vi "DAQ_Controls_Integration.vi"() -> ()   [LabVIEW 2017]
uses:
  <vilib>/MakerHub/LINX/Public/Peripherals/Digital/Digital Write N Chans.vi
  <vilib>/MakerHub/LINX/Private/Local IO/LinxDigitalWrite.vi
  <vilib>/MakerHub/LINX/Public/Utilities/Check Channel.vi
  <vilib>/MakerHub/LINX/Public/Utilities/Open Serial.vi
  <vilib>/MakerHub/LINX/Private/Utilties/Generate Error.vi
  <vilib>/Waveform/WDTOps.llb/WDT Append Waveforms DBL.vi
  <vilib>/MakerHub/LINX/LMH-LINX.lvlib
panel:
  in  "Stop Button":bool
  in  "MANUAL CONTROLS":bool[](array[boolean])
  out "Loop Rate (Hz)":u32
  in  "CHANNELS":u8[](array[numeric])
  in  "Serial Port":refnum<visa-resource-name>
  in  "stop":bool
  out "Waveform Chart":waveform(dbl)(graph)
  in  "Recording Data":bool
  out "Waveform Chart 2":waveform(dbl)(graph)
  out "Numeric":dbl
  out "Numeric 2":dbl
  out "Difference between signals 1 & 2":dbl
  out "Waveform Chart 3":waveform(dbl)(graph)
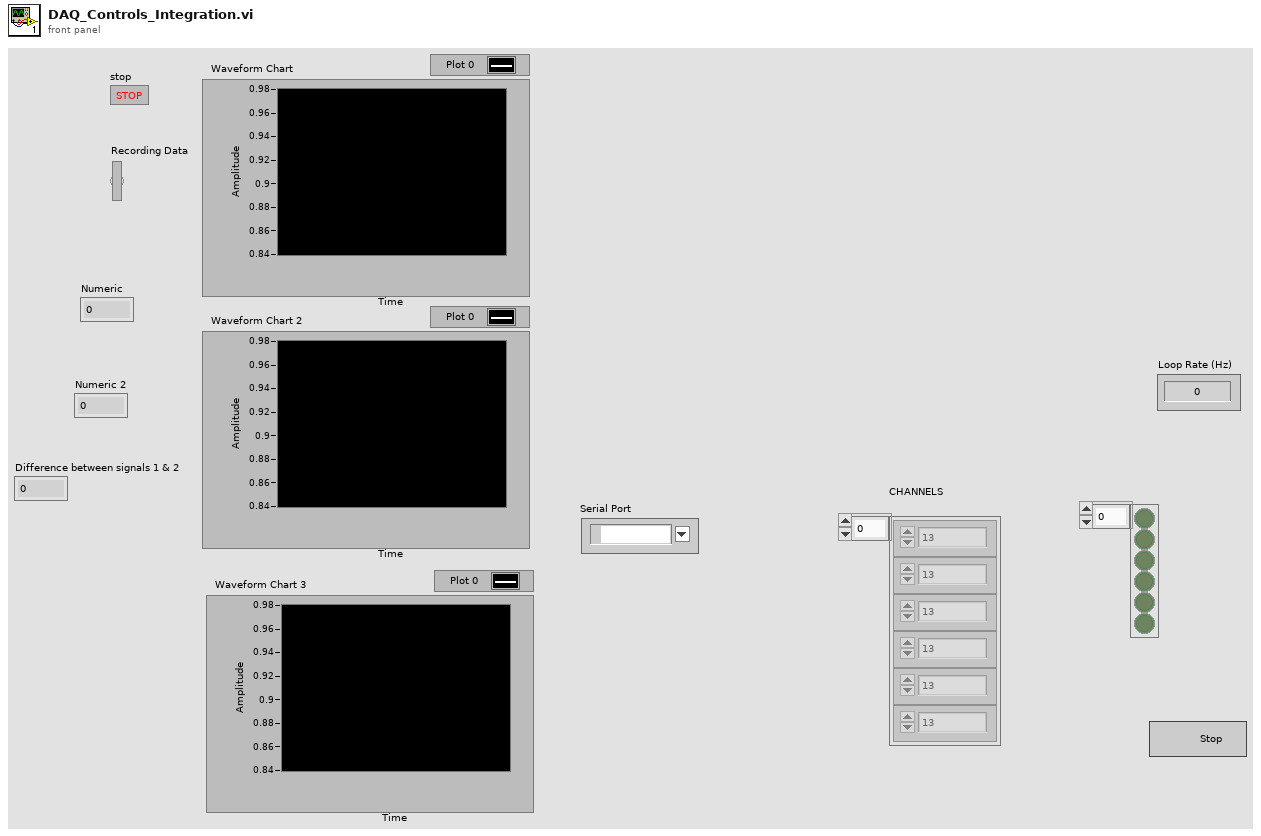
[diagram p1: front panel]
types:
  T1 = typedef "LMH-LINX.lvlib/LINX Ref.ctl" = cluster{"IO":T2, "Interface":T3, "LINX Device Config":T4}
  T2 = typedef "LMH-LINX.lvlib/Platform.ctl" = enum16{"Remote", "Local"}
  T3 = typedef "LMH-LINX.lvlib/Interface.ctl" = enum16{"Serial", "TCP"}
  T4 = typedef "LMH-LINX.lvlib/Device.lvlib/LINX Device Config.ctl" = cluster{"Interface":T3, "COM Port":refnum<visa-resource-name>, "TCP Configuration":T5, "Device Family":u8, "Device ID":u8, "Device Name":string, "TCP Ref":refnum<k5>, "Channels":T6}
  T5 = typedef "LMH-LINX.lvlib/Device.lvlib/TCP Config.ctl" = cluster{"IP Address":string, "Port":u16}
  T6 = typedef "LMH-LINX.lvlib/Channels.ctl" = cluster{"DI":u8[], "DO":u8[], "AI":u8[], "AO":u8[], "PWM":u8[], "QE":u8[], "UART":u8[], "I2C 2":u8[], "SPI":u8[], "CAN":u8[], "Servo":u8[], "AI Ref (V)":dbl, "AI Resolution (Bits)":u8, "AO Ref (V)":dbl, "AO Resolution (Bits)":u8}
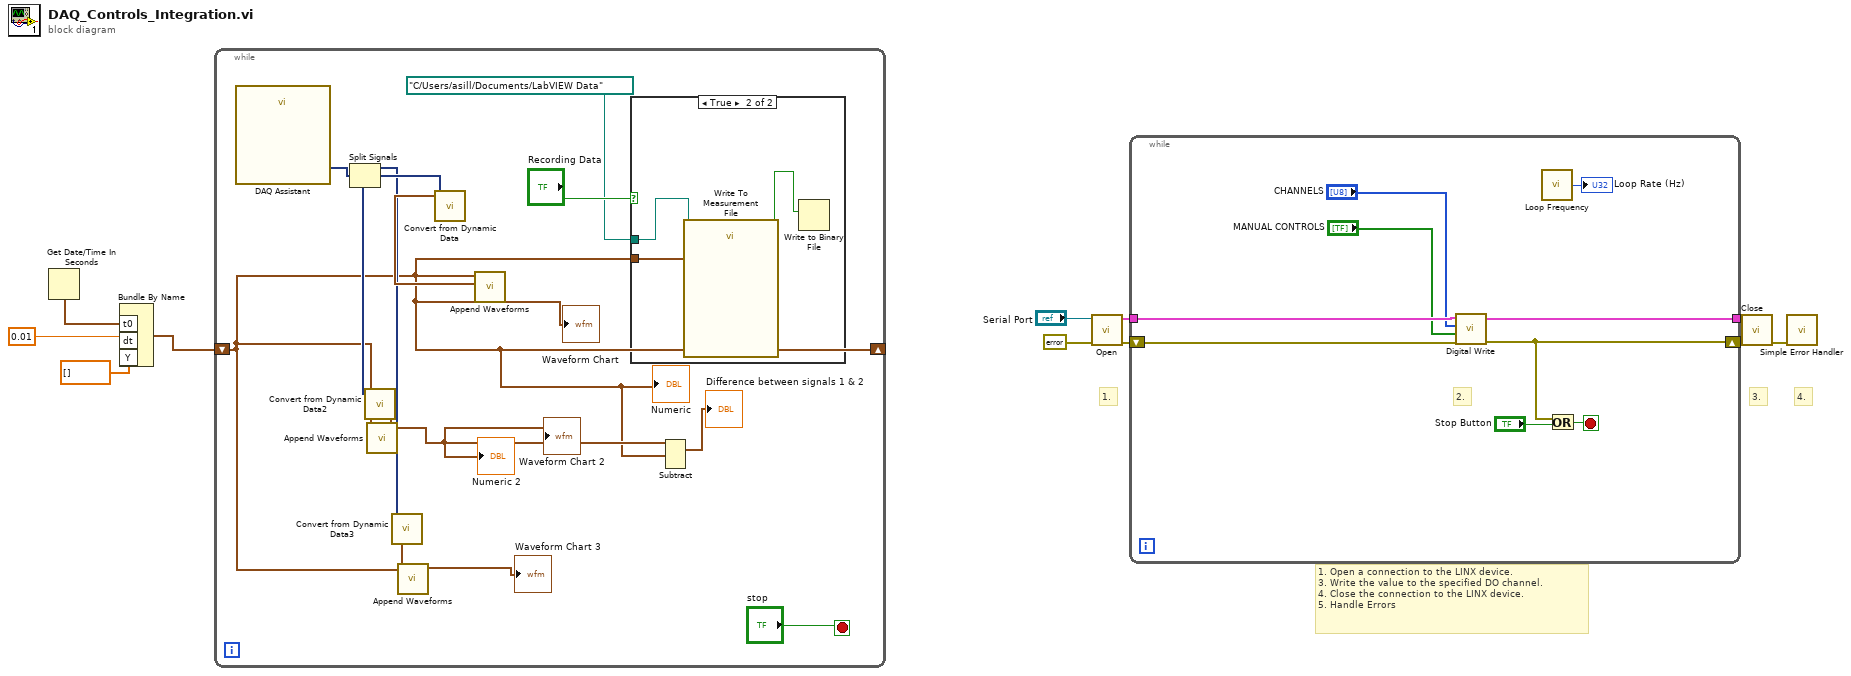
[diagram p0: block diagram]
diagram:
  # "1. Open a connection to the LINX device.\n3. Write the value to the specified DO channel.\n4. Close the connection to the LINX device.\n5. Handle Errors"
  # "4."
  # "3."
  # "1."
  n1 = Get Date/Time In Seconds() -> (seconds since 1Jan1904=w9:timestamp)
  n2 = Bundle By Name("t0"=w9, "dt"=0.01, "Y"=dbl[] []) -> (w10:waveform(dbl))  [unwired: 1 in]
  n3 = while {
    shift-right: [w17] -> _
    shift-left: w10 -> [w13]
    stop <- "stop" stop-if-true
    n4 = call "DAQ Assistant"() -> ("data"=w21:dynamicdata)  [unwired: 16 in, 3 out]
    n5 = Split Signals(w21) -> (w15:dynamicdata, w20:dynamicdata, w19:dynamicdata)  [unwired: 3 in]
    n6 = call "Convert from Dynamic Data2"("Dynamic Data Type"=w19) -> ("Waveform"=w22:waveform(dbl))  [unwired: 3 in]
    n7 = call-poly <vilib>:"Append Waveforms.vi"("waveform B"=w22, "waveform A"=w13) -> ("waveform out"=w18:waveform(dbl))  [unwired: 8 in, 1 out]
    "Waveform Chart 2" <- w18
    "Numeric 2" <- w18
    n8 = call "Convert from Dynamic Data3"("Dynamic Data Type"=w15) -> ("Waveform"=w14:waveform(dbl))  [unwired: 3 in]
    n9 = call-poly <vilib>:"Append Waveforms.vi"("waveform B"=w14, "waveform A"=w13) -> ("waveform out"=→"Waveform Chart 3":waveform(dbl))  [unwired: 8 in, 1 out]
    n10 = call "Convert from Dynamic Data"("Dynamic Data Type"=w20) -> ("Waveform"=w25:waveform(dbl))  [unwired: 3 in]
    n11 = call-poly <vilib>:"Append Waveforms.vi"("waveform B"=w25, "waveform A"=w13) -> ("waveform out"=w17:waveform(dbl))  [unwired: 8 in, 1 out]
    "Waveform Chart" <- w17
    "Numeric" <- w17
    n12 = case shown="True" "Recording Data" {
      tunnel: path "C:/Users/asill/Documents/LabVIEW Data" -> [_ w28]
      tunnel: w17 -> [_ w27]
      frame False {
      }
      frame True {
        n13 = call "Write To Measurement File"("Signals"=w27, "Filename"=w28) -> ("Saving Data"=w29:bool)  [unwired: 15 in, 2 out]
        n14 = Write to Binary File(data=w29) -> ()  [unwired: 5 in, 3 out]
      }
    }
    n15 = Subtract(1:w17, 2:w18) -> (0:→"Difference between signals 1 & 2":waveform(dbl))  [unwired: 1 in, 1 out]
  }
  n16 = call-poly <vilib>:"Open.vi"("Error In"=errorcluster {"status"=FALSE, "code"=0, "source"=""}, "Serial Port"="Serial Port") -> ("Error Out"=w6:errorcluster, "LINX Resource"=w7:T1)  [unwired: 7 in, 1 out]
  n17 = while {
    tunnel: w7 -> [w36]
    tunnel: [w35] -> w5
    shift-right: [w33] -> w4
    shift-left: w6 -> [w34]
    stop <- w38 stop-if-true
    # "2."
    n18 = call-poly <vilib>:"Digital Write.vi"("Error In"=w34, "Values"="MANUAL CONTROLS", "DO Channels"="CHANNELS", "LINX Resource"=w36) -> ("Error Out"=w33:errorcluster, "LINX Resource"=w35:T1)  [unwired: 6 in]
    n19 = call <vilib>:"Loop Frequency.vi"() -> ("Loop Rate (Hz)"=→"Loop Rate (Hz)":u32)
    n20 = Or(x=w33, y="Stop Button") -> (x .or. y?=w38:bool)
  }
  n21 = call <vilib>:"Close.vi"("Error In"=w4, "LINX Resource"=w5) -> ("Error Out"=w2:errorcluster)  [unwired: 9 in]
  n22 = call <vilib>:"Simple Error Handler.vi"("error in (no error)"=w2) -> ()  [unwired: 4 in, 5 out]
